vi "labview_nanonisUDP.vi"(0 "stop":bool) -> ()   [LabVIEW 2019]
uses:
  <userlib>/Nanonis Prog Interface/Nanonis Prog Interface.lvlib
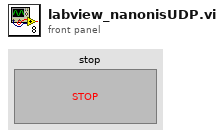
[diagram p1: front panel]
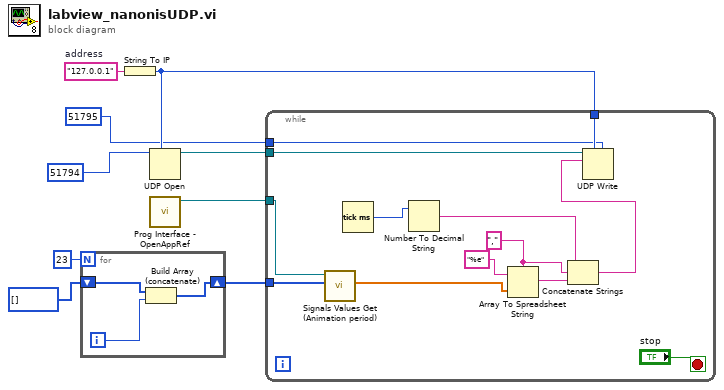
[diagram p0: block diagram]
diagram:
  w4 = "127.0.0.1"  # address
  n1 = for {
    N: 23 -> [_]
    shift-right: [w11] -> w6
    shift-left: i32[] [] -> [w12]
    i -> [w10]
    n2 = Build Array (concatenate)(w12, w10) -> (w11:i32[])
  }
  n3 = String To IP(1:w4) -> (0:w3:u32)
  n4 = UDP Open(7:w3, 11:u16 51794 ("port")) -> (port=w9:refnum<k16>)  [unwired: 3 in, 2 out]
  n5 = call <userlib>:"Prog Interface - OpenAppRef.vi"() -> ("Application reference"=w5:refnum<vi>)  [unwired: 6 in, 1 out]
  n6 = while {
    tunnel: w9 -> [w25]
    tunnel: w6 -> [w24]
    tunnel: w5 -> [w23]
    tunnel: w3 -> [w20]
    tunnel: u16 51795 ("port") -> [w19]
    stop <- "stop" stop-if-true
    w17 = "," ("delimiter (Tab)")
    n7 = call <userlib>:"Signals Values Get (Animation period).vi"("Signals indexes (0-23)"=w24, "Application ref in"=w23) -> ("Signals Values"=w21:sgl[])  [unwired: 6 in, 2 out]
    n8 = Tick Count (ms)() -> (millisecond timer value=w15:u32)
    n9 = Number To Decimal String(number=w15) -> (decimal integer string=w16:string)  [unwired: 1 in]
    n10 = Array To Spreadsheet String(delimiter (Tab)=w17, array=w21, 3:"%e" ("format string")) -> (spreadsheet string=w18:string)
    n11 = Concatenate Strings(w16, w17, w18) -> (w13:string)
    n12 = UDP Write(address=w20, port or service name=w19, connection ID=w25, data in=w13) -> ()  [unwired: 2 in, 2 out]
  }
